vi "Get Error_Window_Behaviour.vi"(8 "error in (no error)":errorcluster, 11 "Settings in":refnum<class "Settings.lvclass">) -> (0 "error out":errorcluster, 2 "Error_Window_Behaviour":T1, 3 "Settings out":refnum<class "Settings.lvclass">)   [LabVIEW 2023, in "Error Manager.lvlib" / "Settings.lvclass"]
uses:
  Settings.lvclass
  Settings.lvclass/Settings.ctl
  Window_Behaviour (enum).ctl
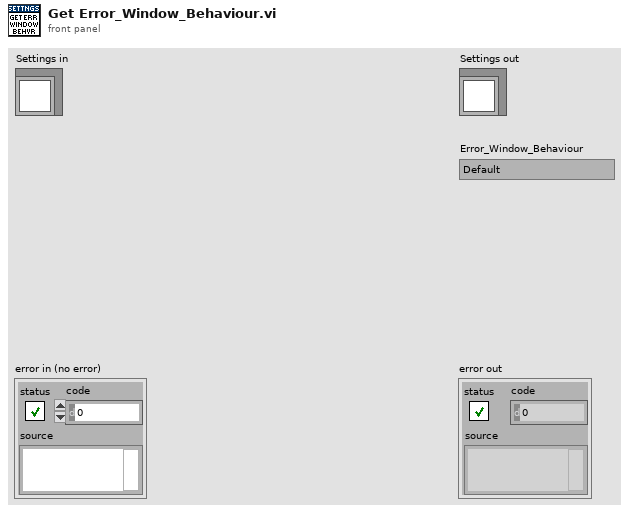
[diagram p1: front panel]
types:
  T1 = typedef "Error Manager.lvlib/Settings.lvclass/Window_Behaviour (enum).ctl" = enum16{"Default", "Floating", "Modal"}
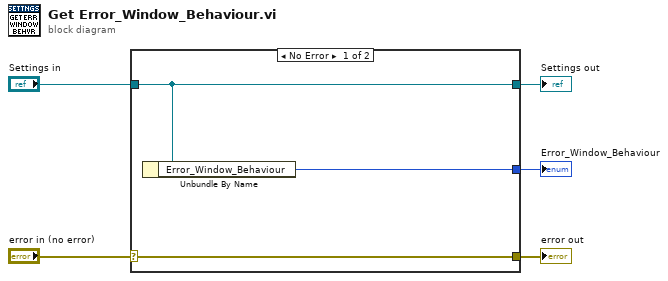
[diagram p0: block diagram]
diagram:
  n1 = case shown="No Error" "error in (no error)" {
    selector: "error in (no error)" -> [w8 w9]
    tunnel: [w8 w9] -> w4
    tunnel: [w7 w10] -> w2
    tunnel: "Settings in" -> [w7 w10]
    tunnel: [w6 _] -> w1
    frame No Error {
      n2 = Unbundle By Name(w7) -> ("Error_Window_Behaviour"=w6:T1)
    }
    frame Error {
    }
  }
  "error out" <- w4
  "Settings out" <- w2
  "Error_Window_Behaviour" <- w1
